vi "popup.vi"() -> ()   [LabVIEW 2014]
doc: "Target VI used in conjunction with the asynchronous call examples."
panel:
  in  "닫기":bool
  out "?":string="ABCDE 1A 절차는 AB(앞 두글자)1A\nCLRD : Cleared\nINTL international\nR/V 레이더벡터\nC/M, D/M \nDep : departure \nApp : approach\nFreq : frequency       \nProb : problem\nSQ : squawk\nP/B : pushback\nE/S : engine start\nRwy : runway\nQ : QNH\nTO : takeoff\nGA : go around\nSay again\n"
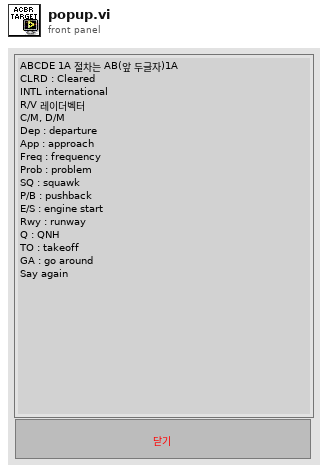
[diagram p1: front panel]
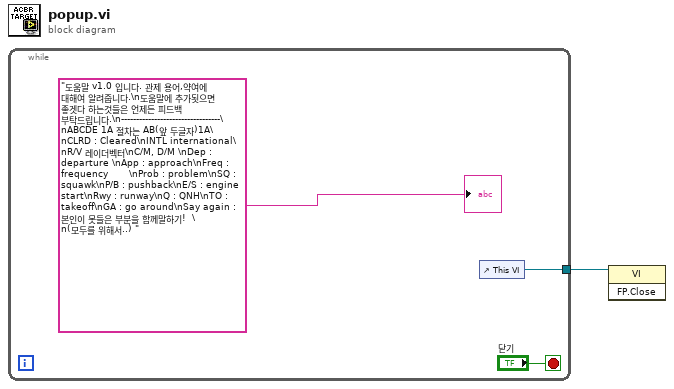
[diagram p0: block diagram]
diagram:
  n1 = while {
    tunnel: [w2] -> w1
    stop <- "닫기" stop-if-true
    n2 = control-ref of="This VI"() -> (w2:refnum<vi>)
    "?" <- "도움말 v1.0 입니다. 관제 용어,약여에 대해여 알려줍니다.\n도움말에 추가됫으면 좋겟다 하는것들은 언제든 피드백 부탁드립니다.\n---------------------------------\nABCDE 1A 절차는 AB(앞 두글자)1A\nCLRD : Cleared\nINTL international\nR/V 레이더벡터\nC/M, D/M \nDep : departure \nApp : approach\nFreq : frequency       \nProb : problem\nSQ : squawk\nP/B : pushback\nE/S : engine start\nRwy : runway\nQ : QNH\nTO : takeoff\nGA : go around\nSay again : 본인이 못들은 부분을 함께말하기!  \n(모두를 위해서..) "
  }
  n3 = invoke class="VI" method="FP.Close"(reference=w1) -> ()  [unwired: 2 in, 3 out]
